vi "SortSensorData.vi"(5 "index_high":i16, 7 "index_low":i16, 8 "error in (no error)":errorcluster, 11 "BME68x in":refnum<class "BME680.lvclass">) -> (0 "error out":errorcluster, 3 "BME68x out":refnum<class "BME680.lvclass">)   [LabVIEW 2022 SP3, in "BME680.lvlib" / "BME680.lvclass"]
uses:
  BME680.lvclass
  BME680.lvclass/BME680.ctl
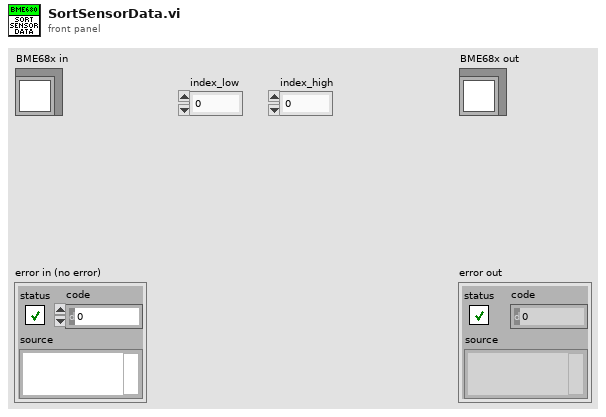
[diagram p1: front panel]
types:
  T1 = typedef "BME680.lvlib/BME680.lvclass/Data.ctl" = cluster{"Status":u8, "GasIdx":u8, "MeasIdx":u8, "ResHeat":u8, "iDac":u8, "GasWait":u8, "Temp":u16, "Pres":u32, "Hum":u8, "Gas Res":u8}
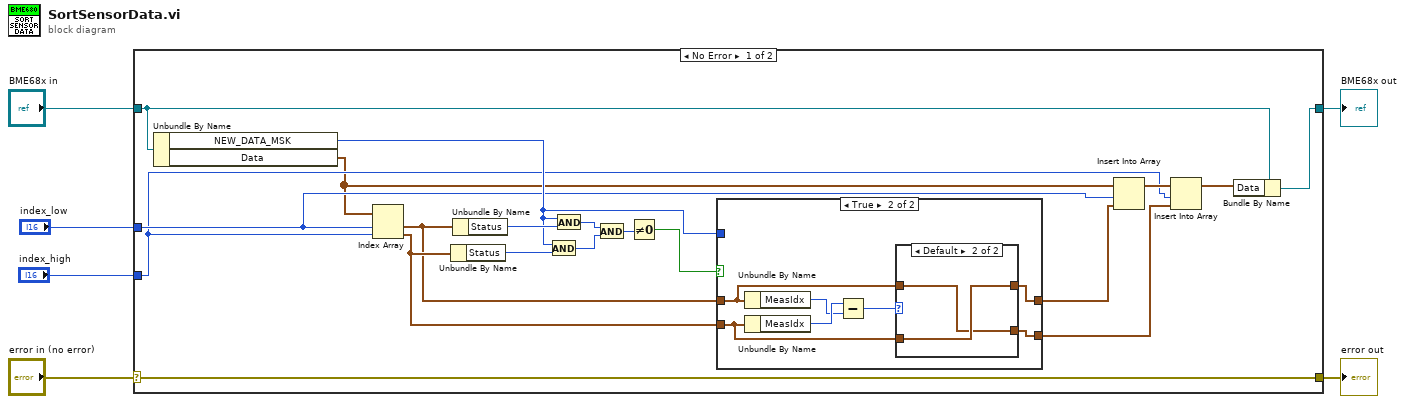
[diagram p0: block diagram]
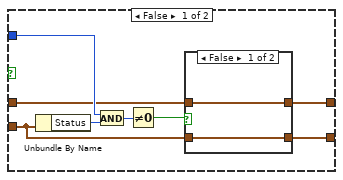
[diagram p2: hidden frame]
diagram:
  n1 = case shown="No Error" "error in (no error)" {
    selector: "error in (no error)" -> [w25 w50]
    tunnel: [w25 w50] -> w5
    tunnel: [w7 w49] -> w3
    tunnel: "BME68x in" -> [w9 w49]
    tunnel: "index_low" -> [w15 _]
    tunnel: "index_high" -> [w12 _]
    frame No Error {
      n2 = Unbundle By Name(w9) -> ("NEW_DATA_MSK"=w16:u8, "Data"=w10:T1[])
      n3 = Index Array(array=w10, index #1=w15, index #2=w12) -> (element #1=w23:T1, element #2=w24:T1)
      n4 = Unbundle By Name(w24) -> ("Status"=w21:u8)
      n5 = Unbundle By Name(w23) -> ("Status"=w22:u8)
      n6 = And(x=w16, y=w21) -> (x .and. y?=w20:u8)
      n7 = And(x=w16, y=w22) -> (x .and. y?=w19:u8)
      n8 = And(x=w19, y=w20) -> (x .and. y?=w18:u8)
      n9 = Not Equal To 0?(x=w18) -> (x != 0?=w17:bool)
      n10 = case shown="True" w17 {
        tunnel: w23 -> [w28 w40]
        tunnel: w24 -> [w29 w41]
        tunnel: w16 -> [w31 _]
        tunnel: [w27 w39] -> w11
        tunnel: [w26 w38] -> w14
        frame False {
          n11 = Unbundle By Name(w29) -> ("Status"=w32:u8)
          n12 = And(x=w31, y=w32) -> (x .and. y?=w33:u8)
          n13 = Not Equal To 0?(x=w33) -> (x != 0?=w30:bool)
          n14 = case shown="False" w30 {
            tunnel: w29 -> [w34 w37]
            tunnel: [w35 w37] -> w26
            tunnel: [w34 w36] -> w27
            tunnel: w28 -> [w35 w36]
            frame False {
            }
            frame True {
            }
          }
        }
        frame True {
          n15 = Unbundle By Name(w40) -> ("MeasIdx"=w43:u8)
          n16 = Unbundle By Name(w41) -> ("MeasIdx"=w44:u8)
          n17 = Subtract(x=w44, y=w43) -> (x-y=w42:u8)
          n18 = case shown="Default" w42 {
            tunnel: [w45 w48] -> w38
            tunnel: w41 -> [w46 w48]
            tunnel: [w46 w47] -> w39
            tunnel: w40 -> [w45 w47]
            frame 0..2 {
            }
            frame Default {
            }
          }
        }
      }
      n19 = Insert Into Array(array=w10, index=w15, new element=w14) -> (w13:T1[])
      n20 = Insert Into Array(array=w13, index=w12, new element=w11) -> (w8:T1[])
      n21 = Bundle By Name(cluster=w9, "Data"=w8) -> (w7:refnum<class "BME680.lvclass">)
    }
    frame Error {
    }
  }
  "error out" <- w5
  "BME68x out" <- w3
